vi "Cria_path_local.vi"(4 "caminho final":string) -> (0 "Saida Path string":string, 2 "Saida Path inteiro":path)   [LabVIEW 2012]
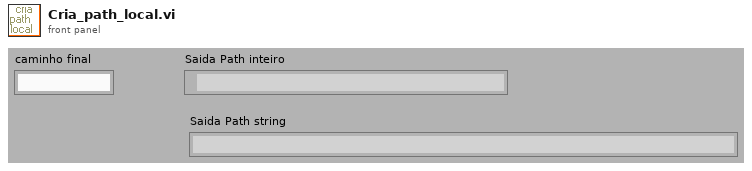
[diagram p1: front panel]
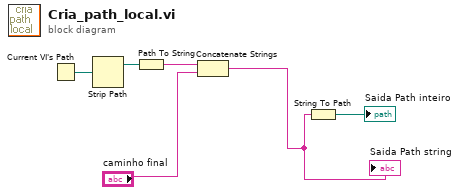
[diagram p0: block diagram]
diagram:
  n1 = Current VI's Path() -> (path=w5:path)
  n2 = Strip Path(path=w5) -> (stripped path=w1:path)  [unwired: 1 out]
  n3 = Path To String(path=w1) -> (string=w4:string)
  n4 = Concatenate Strings(w4, "caminho final") -> (w2:string)
  "Saida Path string" <- w2
  n5 = String To Path(string=w2) -> (path=→"Saida Path inteiro":path)
